vi "Write RFPM Port.vi"(8 "error in (no error)":errorcluster, 10 "RFPM Port":string, 11 "Vector Path in":refnum<class "Vector 18GHz Path.lvclass">) -> (0 "error out":errorcluster, 3 "Vector Path out":refnum<class "Vector 18GHz Path.lvclass">)   [LabVIEW 2023, in "RFFixtureCharact.RFPM.lvlib" / "Vector 18GHz Path.lvclass"]
uses:
  Vector 18GHz Path.lvclass
  Vector 18GHz Path.lvclass/Vector 18GHz Path.ctl
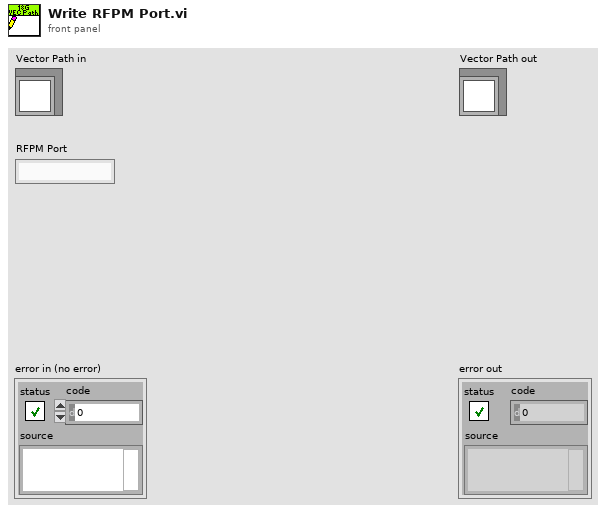
[diagram p1: front panel]
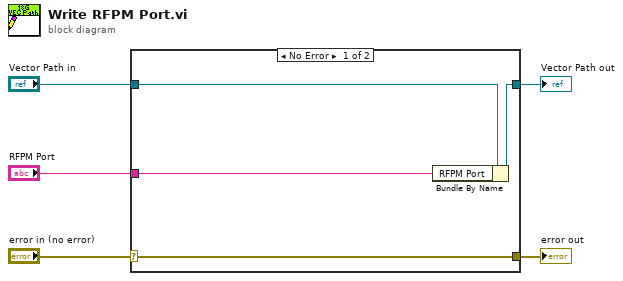
[diagram p0: block diagram]
diagram:
  n1 = case shown="No Error" "error in (no error)" {
    selector: "error in (no error)" -> [w9 w10]
    tunnel: [w9 w10] -> w4
    tunnel: [w7 w11] -> w2
    tunnel: "Vector Path in" -> [w8 w11]
    tunnel: "RFPM Port" -> [w6 _]
    frame No Error {
      n2 = Bundle By Name(cluster=w8, "RFPM Port"=w6) -> (w7:refnum<class "Vector 18GHz Path.lvclass">)
    }
    frame Error {
    }
  }
  "error out" <- w4
  "Vector Path out" <- w2
